vi "AlliGator Calibrated Phasor Maps Series Script.vi"(0 "Alligator Queue Elements in":T2[](array[typedef]), 1 "Calibration Map/Gate Step List":T1[](array[typedef]), 2 "Destination Folder":path, 3 "File Suffix (# Steps will be added)":string caption="File Name (# Steps will be added)", 4 "Save Phasor Plot":bool, 5 "Error In":errorcluster, 6 "Phasor Graph refnum":refnum<vi>) -> (14 "Alligator Queue Elements out":T2[](array[typedef]), 17 "Message":string, 19 "Error Out":errorcluster)   [LabVIEW 2021, in "AlliGator Scripts.lvlib"]
doc: "Loops through a series of FLI Dataset files, loads them with the specified gate step, and performs an All ROIs Phasor Analysis, using the resulting phasor plot as Phasor Calibration Map. This map is then save and optionally, the phasor plot as well."
uses:
  AlliGator Scripts.lvlib
  Action Engine/AlliGator Q Element.ctl
  Action Engine/AlliGator Q Event.ctl
  AlliGator Dataset + Calibration Map + Gate Step.ctl
  Globals, Variables, Constants/AlliGator Variables List.ctl
  Action Engine/Alligator Elements Order in Action Stack.ctl
  Graphs/XY Graph/XY Graph Mouse Click Event Data.ctl
  Graphs/XY Graph/XY Graph Refnum.ctl
  <vilib>/Utility/miscctls.llb/LVPoint32TypeDef.ctl
  Graphs/XY Graph/XY Graph New Plot Name Data.ctl
  Files/Load-Save File Info.ctl
  Action Engine/AlliGator Add Single Action to Stack.vi
  Action Engine/AlliGator Add Action Array to Stack.vi
  Action Engine/AlliGator Action Engine.lvlib
  Strings/Strings.lvlib
  Files/AlliGator Files.lvlib
  Globals, Variables, Constants/AlliGator Globals, Variables & Constants.lvlib
  Graphs/XY Graph/XY Graph Add-Ons.lvlib
  Files/Files.lvlib
panel:
  out "Series Length":i32
  # "see the AlliGator License on the block diagram (Ctrl+E or Window:Show Block Diagram)"
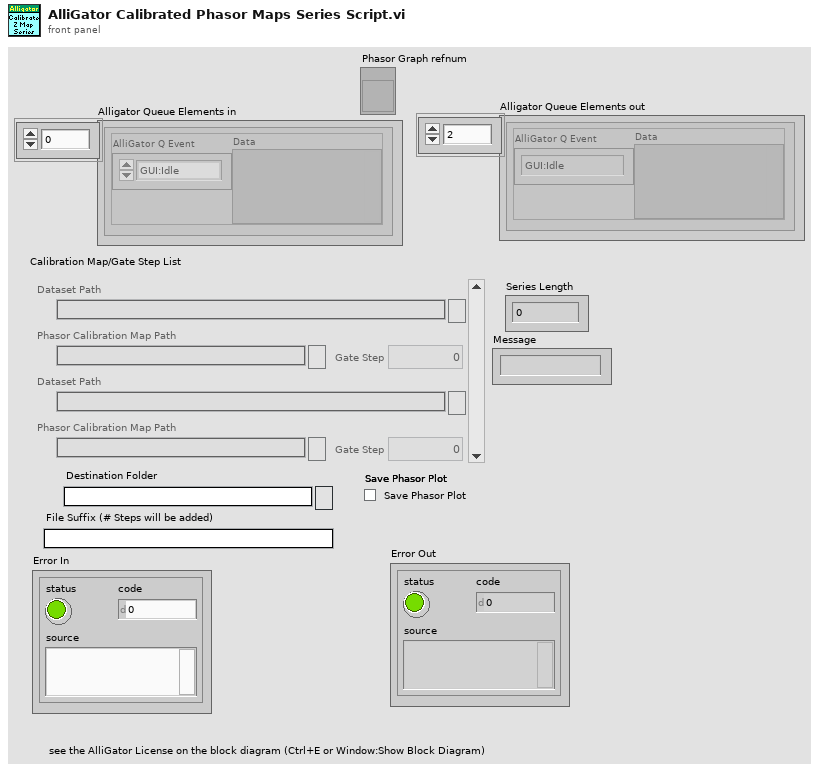
[diagram p1: front panel]
types:
  T1 = typedef "AlliGator Scripts.lvlib/AlliGator Dataset + Calibration Map + Gate Step.ctl" = cluster{"Phasor Calibration Map Path":path, "Gate Step":i32, "Dataset Path":path}
  T2 = typedef "AlliGator Action Engine.lvlib/AlliGator Q Element.ctl" = cluster{"AlliGator Q Event":T3, "Data":variant}
  T3 = typedef "AlliGator Action Engine.lvlib/AlliGator Q Event.ctl" = enum16{"---- Files ----", "Files:Set Batch Export Files To Save", "Files:Set Dataset Loading & Pre-processing Options", "Files:Check #Frames in Dataset", "Files:Increment Frame Index", "Files:Open Mask Image", "Files:Open White Light Image", "Files:Open Single Dataset", "Files:New Folder of Folders Selected", "Files:Load File (all Types)_Scriptable", "Files:Move Flattened Series to Folders Series", "Files:Select Folder", "Files:Load FLI Dataset", "Files:Load Swiss SPAD 1 Dataset", "Files:Load Swiss SPAD 2 Dataset", "Files:Load .sdt FLI Dataset", "Files:Load .ptu FLI Dataset", "Files:Load .bin FLI Dataset", "Files:Load Single Gate Image Folder", "Files:Load I/m/phi Dataset (deprecated)", "Files:Load Single Image", "Files:Subtract Background File", "Files:Export FLI Dataset", "Files:Load HDF5 FLI Dataset", "Files:Set Destination File Path", "Files:Save Mask Image", "Files:Batch Conversion", "Files:New Folder Selected", "Files:Close FLI Dataset", "Files:Close FLI Dataset Series", "Files:Close White Light Image", "Files:Close Mask Image", "---- FLI Dataset ----", "FLI Dataset:Channel Arithmetic", "FLI Dataset:Export Average Lifetime Map as ASCII", "FLI Dataset:Export User-Defined Quantity Map as ASCII", "FLI Dataset:Python Function FLI Dataset Event", "FLI Dataset:ROI Analysis", "FLI Dataset:Tilted Logistic Square Gated IRF Characteristics Map", "FLI Dataset:Logistic Square Gated IRF Characteristics Map", "FLI Dataset:Square Gated IRF Characteristics Map", "FLI Dataset:Multi-ROI Single-Pixel Phasor Analysis", "FLI Dataset:Multi-ROI Single-Pixel NLSF Analysis", "FLI Dataset:All ROIs IRF Extraction", "FLI Dataset:All ROIs Decay Fit Non-Interactive (Fast + Individual IRF)", "FLI Dataset:All ROIs Phasor Analysis", "FLI Dataset:All ROIs Decay Fit", "FLI Dataset:Fluorescence Decay Statistics", "FLI Dataset:Update Decay Statistics Graph", "FLI Dataset:Get Decay from ROI", "FLI Dataset:All ROIs Average Lifetimes", "---- FLI Dataset Series ----", "FLI Dataset Series:Sum All Datasets in Series", "FLI Dataset Series:Add Dataset to Accumulated Dataset", "FLI Dataset Series:Display Accumulated Dataset", "FLI Dataset Series:Clear Dataset Series Sum", "FLI Dataset Series:Time-Series Analysis (NLSF)", "FLI Dataset Series:Time-Series Analysis (Phasor)", "---- Image ----", "Image:Update Image Profile Plots", "Image:Image Histogram Cursor Move", "Image:Image Histogram", "Image:Image Contrast", "Image:Set Image Histogram Cursor Move Flag", "Image:Clear Image Overlay", "Image:Use ROI as Search Area", "Image:Set ROI Diameter", "Image:Save Image Data as TIFF", "Image:Save Displayed Image with Overlay", "Image:Save Image Overlay Only", "Image:Save Image as Hot Pixel Mask", "Image:Change Source Image Color Palette", "Image:Copy Image to Clipboard", "Image:Source Image ROI Selection", "Image:Delete All ROIs", "Image:Delete All Unselected ROIs", "Image:Delete ROI", "Image:Merge All ROIs", "Image:Store ROI", "Image:Source Image ROI Storage", "Image:Export ROI Description to Notebook", "Image:Save ROI", "Image:Load ROI", "Image:Paste ROI Definition", "Image:Clear ROI", "Image:Identify ROIs in Mask Image", "Image:Create Complementary ROI", "Image:Create Contour ROI", "Image:Create ROI(s) from Pixels with Peak above Min_Scriptable", "Image:Create ROI(s) from Pixels with Intensity above Min_Scriptable", "Image:Compute ROI Statistics", "Image:Delete ROI(s) based on ROI Characteristics", "Image:Create ROI Grid", "Image:ROI to Individual Pixel ROIs", "Image:Python Function Source Image Event", "Image:Show Phasor Calibration Map ROI Centers", "Image:Convert ROI to Mask Image", "Image:Mouse Move", "Image:Mouse Up", "Image:Set Source Image Mouse Move Flag", "Image:Add Scale Bar Overlay", "Image:Delete Existing ROIs Option", "Image:Overlay ROI Median", "Image:Check Current ROI", "---- Decay ----", "Decay:Clear IRF/Reference Plot", "Decay:Clear Local IRFs", "Decay:Add Decay to Graph", "Decay:Smoothen Plot", "Decay:Smoothen Plot Tail", "Decay:Average Selected Plots", "Decay:Extract IRF", "Decay:Optimal IRF Extraction", "Decay:Threshold IRF", "Decay:Fit to Model IRF", "Decay:Fit IRF to Square Gate", "Decay:Fit IRF to Logistic Square Gate", "Decay:Fit IRF to Tilted Logistic Square Gate", "Decay:Create Bounding Cursors Set", "Decay:Export Bounding Cursors Definition to Notebook", "Decay:Denoise Plot", "Decay:Compute Cumulative Function", "Decay:Use as Reference Decay", "Decay:Show Reference Decay/IRF", "Decay:Extrapolate Decay", "Decay:Create Head & Tail Bounding Cursors", "Decay:Store Cursor-defined Head & Tail Fractions", "Decay:Rebin Plot", "Decay:1-Normalize Decay", "Decay:[0-1]-Normalize Plot", "Decay:Straighten Decay", "Decay:Shift Decay", "Decay:Fold Decay", "Decay:Fit Decay", "Decay:Global Fit of Selected Decays", "Decay:Post Global Fit Script", "Decay:Add Global Fit Parameters to Graph", "Decay:Add Decay Parameter(s) to Plot (Graph)", "Decay:Export Decay to Phasor Graph", "Decay:Plot Decay Shifts", "Decay:Compute Average Lifetime", "Decay:Plot Convolution", "Decay:Graph Tip Strip Update", "---- Decay Statistics ----", "Decay Statistics:Tip Strip Update", "---- Intensity Time Trace ----", "Intensity Time Trace:Use File Timestamp", "Intensity Time Trace:Load Intensity Corrections File", "Intensity Time Trace:Clear Intensity Corrections File", "Intensity Time Trace:Tip Strip Update", "---- Phasor Plot ----", "Phasor Plot:Build Phasor Plot", "Phasor Plot:Change Phasor Plot Color Palette", "Phasor Plot:Adjust Phasor Plot Display Range", "Phasor Plot:Highlight Image ROI in Phasor Plot", "Phasor Plot:Save Phasor Plot Image with Overlay", "Phasor Plot:Export Complex Phasor Map", "Phasor Plot:Export Phasor Ratio Map", "Phasor Plot:Export Average Lifetime Map", "Phasor Plot:Compute Phase Lifetime Histogram", "Phasor Plot:Compute Phasor Ratio Histogram", "Phasor Plot:Compute Phase Lifetime vs Intensity Scatter Plot", "Phasor Plot:Weber 2-Component Decomposition", "Phasor Plot:Update Phasor Color Map Vertices", "Phasor Plot:Clear Phasor Overlay", "Phasor Plot:Use Segment Extremities as References", "Phasor Plot:Use UC/Segment Intersections as References", "Phasor Plot:Use UC/Principal Axis Intersections as References", "Phasor Plot:Use UC/Linear Fit Intersections as References", "Phasor Plot:Update Phasor Plot Reference", "Phasor Plot:Show Local Phasor Info in Phasor Plot", "Phasor Plot:Update Phasor Plot State", "Phasor Plot:Phasor Plot ROI Storage", "Phasor Plot:Phasor Plot ROI Selection", "Phasor Plot:Python Function Phasor Plot Event", "Phasor Plot:Overlay Phasor ROI, Ratio or Map in Source Image", "Phasor Plot:Compute Decay of Selected Phasors", "Phasor Plot:Phasor at Image Pixel", "Phasor Plot:Mouse Move", "Phasor Plot:Mouse Up", "Phasor Plot:Display Range Mouse Move", "Phasor Plot:Set Mouse Move Flag", "---- Phasor Graph ----", "Phasor Graph:Calibrated Phasor Map Series", "Phasor Graph:Whole Image Phasor Scatter Plot (deprecated)", "Phasor Graph:Get Phasor Value", "Phasor Graph:Create New Phasor Plot Dialog", "Phasor Graph:Update Last Phasor Value", "Phasor Graph:Update Phasor (m, phi)", "Phasor Graph:Remove Single Phasor from Plot", "Phasor Graph:Add Single Phasor to Plot", "Phasor Graph:Remove Phasor Plot", "Phasor Graph:Remove Selected Phasor Plots", "Phasor Graph:Clear Phasor Data", "Phasor Graph:Clear Phasor Graph", "Phasor Graph:Cursor Move", "Phasor Graph:Draw Cursor Connecting Line", "Phasor Graph:Clear Cursor Connecting Line", "Phasor Graph:Find UC Intersection", "Phasor Graph:Use UC/Cursor-Defined Line Intersections", "Phasor Graph:Use Selected Plots Fitted Line/UC Intersections", "Phasor Graph:Use Selected Plots Principal Axis/UC Intersections", "Phasor Graph:Show Single Phasor", "Phasor Graph:Save Single Phasor Plot", "Phasor Graph:Save All Phasor Plots", "Phasor Graph:Load Phasor Plot(s)", "Phasor Graph:Phasor Multiplication", "Phasor Graph:Compute Average Phasor", "Phasor Graph:Compute Multiple Average Phasors (Selected Plots)", "Phasor Graph:Export Single Phasor Plot Phase Lifetimes", "Phasor Graph:Phase Lifetime Trajectory", "Phasor Graph:Phase Lifetime vs Intensity Scatter Plot (deprecated)", "Phasor Graph:Parameter 2 vs Parameter 1 Scatter Plot", "Phasor Graph:Use Cursor n Location", "Phasor Graph:Set Reference n to Current Phase Lifetime Value", "Phasor Graph:Set Reference n to Lifetime Value", "Phasor Graph:Set Cursor n Location", "Phasor Graph:Save Phasor Graph Image", "Phasor Graph:Update SEPL Plot", "Phasor Graph:Export Single Phasor Plot Data", "Phasor Graph:Export Selected Phasor Plots Data", "Phasor Graph:Python Function Phasor Graph Event", "Phasor Graph:Tip Strip Update", "---- Calibration ----", "Calibration:Set Calibration Type", "Calibration:Load/Save Phasor Calibration", "Calibration:Load/Save Phasor Calibration Series", "Calibration:Load/Save Phasor Calibration Map", "Calibration:Use as Calibration", "Calibration:Compute Optimal Calibration from Phasor References", "Calibration:Clear Phasor Calibration", "Calibration:Single Phasor Calibration Information", "Calibration:Use as Calibration Series", "Calibration:Use as Calibration Map", "Calibration:Clear Calibration Series", "Calibration:Phasor Calibration Series Information", "Calibration:Clear Calibration Map", "Calibration:Phasor Calibration Map Information", "Calibration:Apply Phasor Calibration", "Calibration:Update Single Plot Calibration", "Calibration:Update Multiple Plots Calibration", "Calibration:Clear Single Plot Calibration", "Calibration:Clear All Plots Calibrations", "Calibration:Clear Plot(s) Calibration(s)?", "Calibration:Phasor Calibration Maps (# Gates Series)", "---- Phasor Ratio ----", "Phasor Ratio:Clear Reference n", "Phasor Ratio:Toggle Selected Plot(s)  Lock to Reference 1", "Phasor Ratio:Use as Reference n", "Phasor Ratio:Send Reference n to Notebook", "Phasor Ratio:Toggle Selected Plot(s)  Lock to Reference 2", "Phasor Ratio:Compute Phasor Ratio at Mouse Location", "Phasor Ratio:Compute Phasor Plot's Average Phasor Ratio", "Phasor Ratio:Compute Time-Series Phasor Ratios", "Phasor Ratio:Fit Line to Phasor Ratio Plot", "Phasor Ratio:Save References", "Phasor Ratio:Load References", "Phasor Ratio:Update Phasor Reference 1", "Phasor Ratio:Update Phasor Reference 2", "Phasor Ratio:Move Cursor n to Reference n", "Phasor Ratio:Use as Phasor Reference 1 Lifetime", "Phasor Ratio:Use as Phasor Reference 2 Lifetime", "Phasor Ratio:Export Phasor Ratio Map as ASCII", "Phasor Ratio:Tip Strip Update", "---- Lifetime & Other Parameters Graph ----", "Lifetime:Tip Strip Update", "---- Decay Fit Parameter Map ----", "Decay Fit Parameter Map:Export ROI NLSF Data as ASCII", "Decay Fit Parameter Map:Set Decay Fit Parameter Map Selection", "Decay Fit Parameter Map:Build Decay Fit Parameter Map", "Decay Fit Parameter Map:Change Decay Fit Parameter Map Color Palette", "Decay Fit Parameter Map:Export Decay Fit Parameter Map Data as ASCII", "Decay Fit Parameter Map:Export All Decay Fit Parameter Maps Data as ASCII", "Decay Fit Parameter Map:Selected Parameter Scatterplot", "Decay Fit Parameter Map:Parameter 2 vs Parameter 1 Scatterplot", "Decay Fit Parameter Map:Save Decay Fit Parameter Map Image", "Decay Fit Parameter Map:Save-Load IRFs & Fit Data", "Decay Fit Parameter Map:Update Local Decay Plots", "Decay Fit Parameter Map:Python Function Decay Fit Parameters Map Event", "Decay Fit Parameter Map:Overlay Decay Fit Parameter Map in Source Image", "Decay Fit Parameter Map:Selected Parameter vs Intensity Scatterplot", "Decay Fit Parameter Map:Mouse Up", "Decay Fit Parameter Map:Display Range Mouse Move", "---- Parameter Map ----", "Parameter Map:Export ROI Parameters Data as ASCII", "Parameter Map:Delete Parameter Map Set", "Parameter Map:Update Parameter List", "Parameter Map:Build Parameter Map", "Parameter Map:Change Parameter Map Color Palette", "Parameter Map:Export Parameter Map Data as ASCII", "Parameter Map:Export All Parameter Maps Data as ASCII", "Parameter Map:Selected Parameter Scatterplot", "Parameter Map:Parameter 2 vs Parameter 1 Scatterplot", "Parameter Map:Selected Parameter vs Intensity Scatterplot", "Parameter Map:Save Parameter Map Image", "Parameter Map:Save-Load IRFs & Parameter Maps (TODO)", "Parameter Map:Set Parameter Map Selection", "Parameter Map:Python Function Parameter Map Event", "Parameter Map:Overlay Parameter Map in Source Image", "Parameter Map:Update Local Decay Plots", "Parameter Map:Mouse Up", "Parameter Map:Display Range Mouse Move", "---- Generic Graph ----", "Generic Graph:Generic XY Graph Event", "Generic Graph:Python Function XY Graph Event", "Generic Graph:New Plot", "Generic Graph:Save Plot", "Generic Graph:XY Plot Histogram", "Generic Graph:Set XY Graph Plot Name", "Generic Graph:Set Last Cursor Style", "Generic Graph:Tip Strip Update", "---- GUI ----", "GUI:Start Script", "GUI:Type of Displayed Image Changed", "GUI:Gate Image Slide Changed", "GUI:Show Busy Icon", "GUI:Show Busy Icon & Abort Button", "GUI:Hide Busy Icon", "GUI:Hide Busy Icon & Abort Button", "GUI:Abort", "GUI:End Script", "GUI:Start Timing", "GUI:End Timing", "GUI:Set State Indicator", "GUI:Send Parameters JSON Strings to Clipboard", "GUI:Set Gate Step", "GUI:Idle", "GUI:Initialization", "GUI:Quit", "GUI:Increment Dataset Index", "GUI:Set Dataset Index to -1", "GUI:Time Series Slider Moved", "GUI:Time Series Slider Changed", "GUI:Toggle Playback or Loop", "GUI:Playback Script", "GUI:Set Phasor Frequency", "GUI:Open Window", "GUI:Start Test Script", "GUI:End Test Script", "DEBUG"}
  T4 = typedef "AlliGator Globals, Variables & Constants.lvlib/AlliGator Variables List.ctl" = enum16{"---- GUI ----", "GUI:Initialization Status", "GUI:State Indicators Refnum", "GUI:Original AlliGator Menu Items", "GUI:Current Action Loop State", "GUI:Script in progress", "GUI:Playback", "GUI:Loop Playback", "GUI:Search ROI Used", "GUI:Search ROI", "Decay Graph Max Legend Size", "Intensity Graph Max Legend Size", "Decay Statistics Graph Max Legend Size", "Phasor Graph Max Legend Size", "Phasor Ratio Graph Max Legend Size", "Lifetime Graph Max Legend Size", "---- Files ----", "Files:Export Dataset Frames as Individual Files", "Files:Show Batch Export Help Balloons", "Files:Frames in Dataset", "Files:ptu File Frame Start Indices", "Files:Current Frame in Dataset", "Files:Current Frame Timestamp", "Files:Dataset Loaded", "Files:Dataset Metadata", "Files:Dataset Channel", "Files:Dataset Data Description", "Files:Background Dataset Metadata", "Files:Background Dataset Channel", "Files:Background Dataset Data Description", "Files:Background File Subtraction", "Files:Background File Path", "Files:Background File Pile-up Correction", "Files:Background File Pixel Well Capacity", "Files:Background File Scaling Factor", "Files:Current Dataset Load Settings", "Files:Dataset Path", "Files:ICCD-specific Information", "Files:Macrotime Gate Separation", "------ Python Plugins ------", "Python Plugins:Information", "Python Plugins:Python Session", "Python Plugins:Valid Python Session?", "---- Source Image ----", "Source Image:ROIs", "Source Image:Current ROI", "Source Image:ROI Event Refnum", "X_Source Image Display Range", "X_Source Image Palette Information", "X_Type of Displayed Image", "X_Time Gate Slider", "Source Image:Palette List", "Source Image:Scale", "Source Image:ROI Overlay Color", "Source Image:Overlay to Erase", "Source Image:Is Displayed Image Accumulated", "Source Image:White Light Image Modified", "Source Image:Mask Image Modified", "---- Image Profile Window ----", "Image Profile:Window Event Refnum", "Image Profile:IntensityType", "Image Profile:Intensity Average Type", "Image Profile:Intensity-weighted SDV", "Image Profile:Box Profile Type", "Image Profile:Window Open", "Image Profile:Plotted Fit Parameter", "------ Phasor Graph -------", "Phasor Graph:Show Line", "---- Phasor Plot ---", "Phasor Plot:Parameters Changed", "Phasor Plot:FLI Dataset Modified since last Calculation", "Phasor Harmonics Data", "Selected Phasor Harmonics", "Phasor Harmonic Manager Event Refnum", "Phasor Plot:ROIs", "Phasor Plot:Current ROI", "Phasor Plot:ROI Event Refnum", "Phasor Plot:Image Reference Points", "Phasor Plot:Computed", "Phasor Plot:Palette Information", "Phasor Plot:Palette List", "Phasor Plot:Phasor Ratio Palette Information", "Phasor Plot:Phasor Ratio Palette List", "Phasor Plot:Image Scale", "Phasor Plot:Image Overlay to Erase", "Phasor Plot:Image Elements to Update", "Phasor Plot:Current Calculation Parameters", "Phasor Plot:Current Calibration Options", "Phasor Plot:Reset Cumulated Phasor Plot", "Phasor Plot:Reference 1", "Phasor Plot:Lifetime Reference 1", "Phasor Plot:Reference 1 Frequency", "Phasor Plot:Reference 2", "Phasor Plot:Lifetime Reference 2", "Phasor Plot:Reference 2 Frequency", "---- Decay Analysis ----", "Number of Selected Decays to Fit", "LS Fit Results", "LAR Fit Results", "BS Fit Results", "Last Decay Max - Min", "Best Fit Parameters", "Best Fit Parameter Names", "Actual Size X", "Actual Size Y", "Binning X", "Binning Y", "Actual # Gates", "Dataset Number", "Gates to...", "Gates Skipped", "Gates to keep", "Gate Step", "Gate Separation", "Reversed Gates", "Pile-up Correction", "Pixel Well Capacity", "Background Subtracted", "Background Subtraction Method", "Background Definition Range", "Background File (deprecated)", "Number of Dataset Accumulated", "Array of Accumulated Dataset Paths", "Do Averaged Datasets", "Destination File Path", "Process Plot Target", "Use 1/D as Phasor Frequency", "---- Decay Fit Parameter Map -----", "Decay Fit Parameter Map:Palette Information", "Decay Fit Parameter Map:Palette List", "---- Parameter Map ----", "Parameter Map:Palette Information", "Parameter Map:Palette List", "------- Local Decay Window ---------", "Local Decay Graph Window:Event Refnum", "Local Decay Graph Window:Use normalized IRF for convolution", "----- Miscellaneous ----", "Misc:Skippable Dialog Windows Status"}
  T5 = enum16{"Start Script", "Load & Analyze Data", "End Script"}
  T6 = typedef "AlliGator Action Engine.lvlib/Alligator Elements Order in Action Stack.ctl" = enum16{"Enqueue 2 AFTER 1", "Enqueue 2 BEFORE 1"}
  T7 = typedef "Files.lvlib/Load-Save File Info.ctl" = cluster{"Load/Save":bool, "File Path":path}
  T8 = typedef "XY Graph Add-Ons.lvlib/XY Graph New Plot Name Data.ctl" = cluster{"XY Graph Refnum":T9, "Plot Index":i32, "Plot Name":string, "Allow Duplicate":bool}
  T9 = typedef "XY Graph Add-Ons.lvlib/XY Graph Refnum.ctl" = refnum<vi>
  T10 = typedef "XY Graph Add-Ons.lvlib/XY Graph Mouse Click Event Data.ctl" = cluster{"Multiplot XY Graph":T9, "Mouse Coordinates":T11}
  T11 = typedef "LVPoint32TypeDef.ctl" = cluster{"Horizontal":i32, "Vertical":i32}
  T12 = cluster{"Mouse Click Event Data":T10, "Save as...":bool}
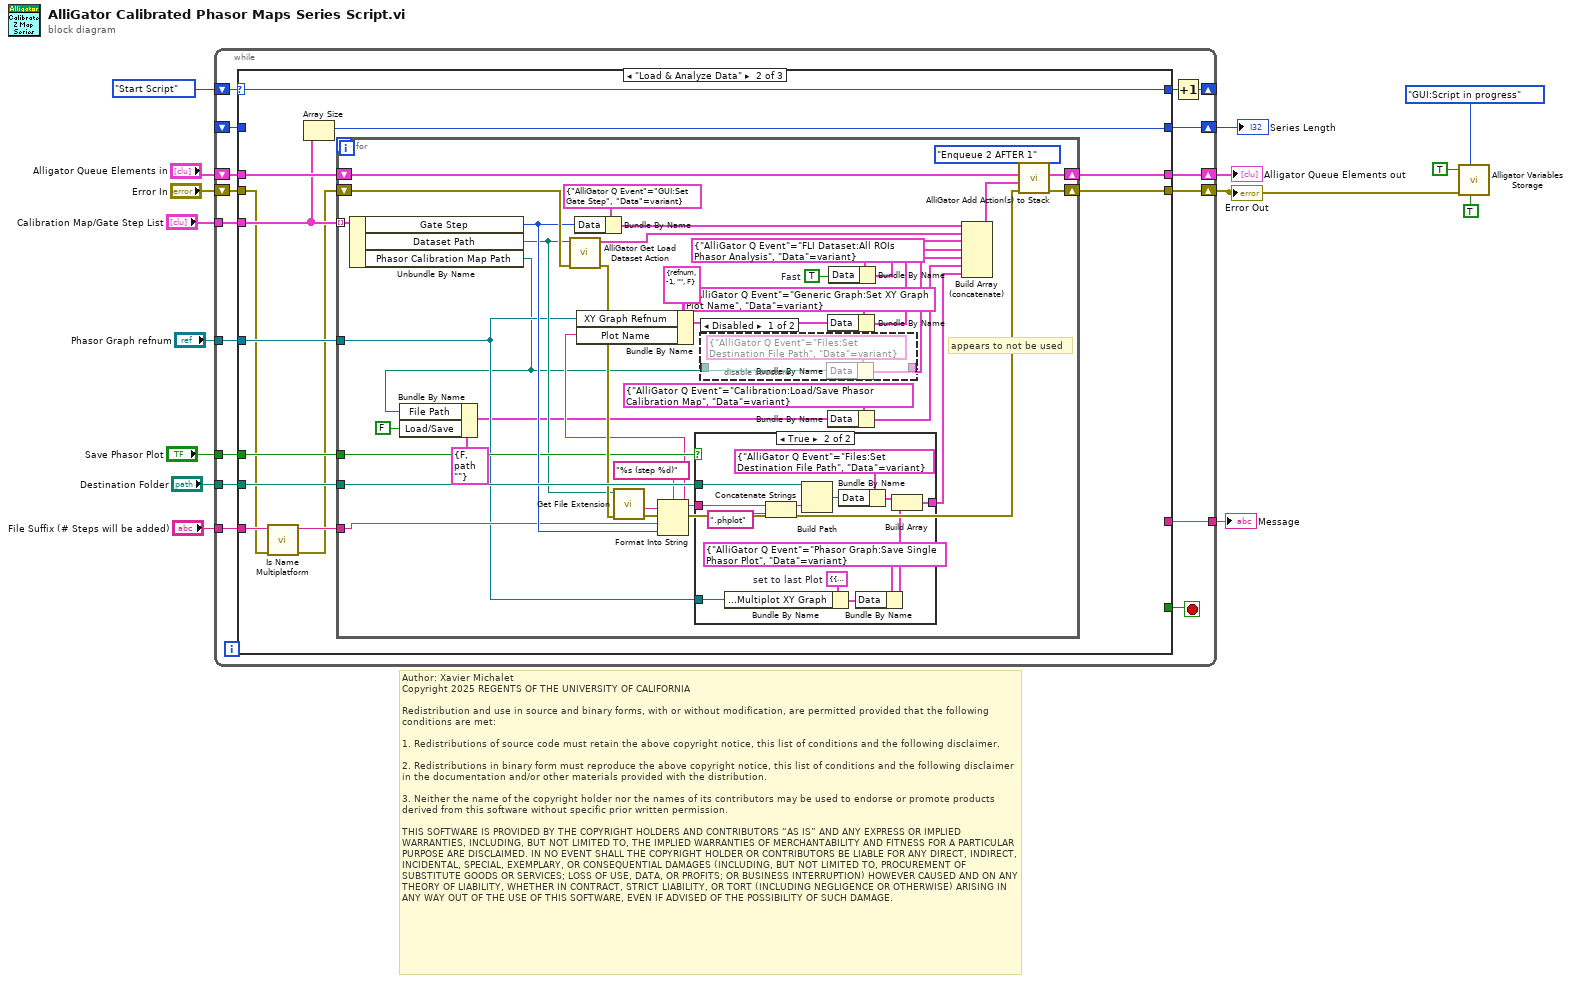
[diagram p0: block diagram]
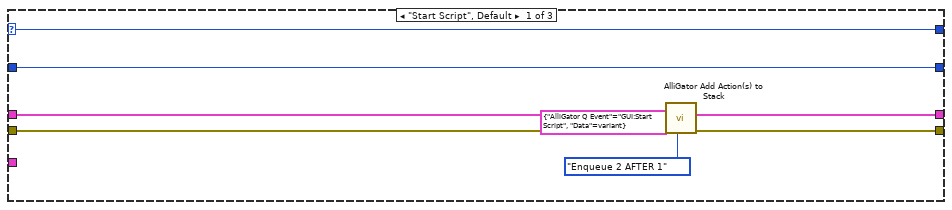
[diagram p2: hidden frame]
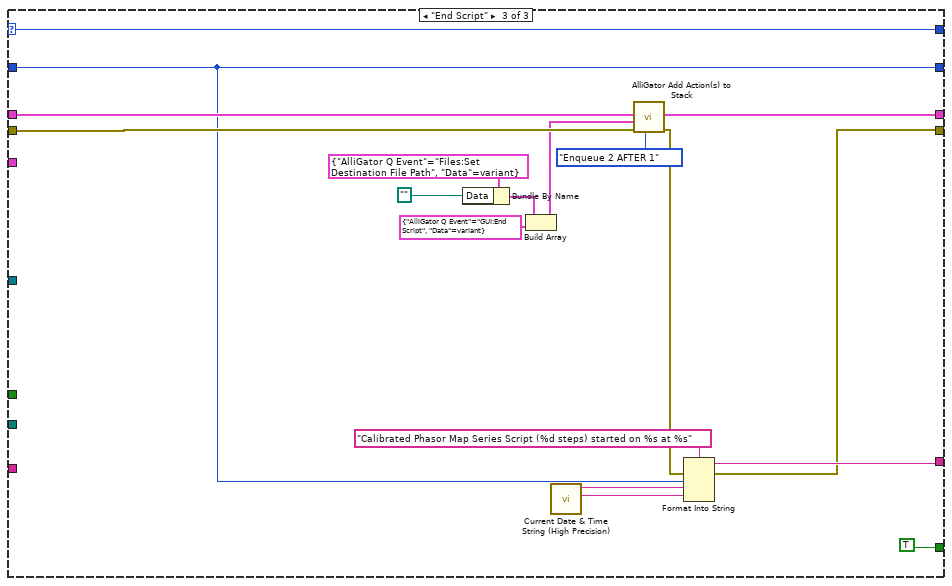
[diagram p5: hidden frame]
diagram:
  # "Author: Xavier Michalet\nCopyright 2025 REGENTS OF THE UNIVERSITY OF CALIFORNIA\n\nRedistribution and use in source and binary forms, with or without modification, are permitted provided that the following conditions are met:\n\n1. Redistributions of source code must retain the above copyright notice, this list of conditions and the following disclaimer.\n\n2. Redistributions in binary form must reproduce the above copyright notice, this list of conditions and the following disclaimer in the documentation and/or other materials provided with the distribution.\n\n3. Neither the name of the copyright holder nor the names of its contributors may be used to endorse or promote products derived from this software without specific prior written permission.\n\nTHIS SOFTWARE IS PROVIDED BY THE COPYRIGHT HOLDERS AND CONTRIBUTORS “AS IS” AND ANY EXPRESS OR IMPLIED WARRANTIES, INCLUDING, BUT NOT LIMITED TO, THE IMPLIED WARRANTIES OF MERCHANTABILITY AND FITNESS FOR A PARTICULAR PURPOSE ARE DISCLAIMED. IN NO EVENT SHALL THE COPYRIGHT HOLDER OR CONTRIBUTORS BE LIABLE FOR ANY DIRECT, INDIRECT, INCIDENTAL, SPECIAL, EXEMPLARY, OR CONSEQUENTIAL DAMAGES (INCLUDING, BUT NOT LIMITED TO, PROCUREMENT OF SUBSTITUTE GOODS OR SERVICES; LOSS OF USE, DATA, OR PROFITS; OR BUSINESS INTERRUPTION) HOWEVER CAUSED AND ON ANY THEORY OF LIABILITY, WHETHER IN CONTRACT, STRICT LIABILITY, OR TORT (INCLUDING NEGLIGENCE OR OTHERWISE) ARISING IN ANY WAY OUT OF THE USE OF THIS SOFTWARE, EVEN IF ADVISED OF THE POSSIBILITY OF SUCH DAMAGE."
  n1 = while {
    shift-right: [w28] -> w6
    shift-left: "Error In" -> [w31]
    shift-right: [w26] -> _
    shift-left: T5."Start Script" -> [w29]
    shift-right: [w24] -> w12
    shift-left: "Alligator Queue Elements in" -> [w30]
    tunnel: "Calibration Map/Gate Step List" -> [w23]
    tunnel: "Destination Folder" -> [w22]
    tunnel: "File Suffix (# Steps will be added)" -> [w21]
    shift-right: [w20] -> w9
    shift-left: _ -> [w19]
    tunnel: "Phasor Graph refnum" -> [w18]
    tunnel: "Save Phasor Plot" -> [w17]
    tunnel: [w16] -> w1
    stop <- w25 stop-if-true
    n2 = case shown="\"Load & Analyze Data\"" w29 {
      selector: w29 -> [w39 w51 w122]
      tunnel: w31 -> [w36 w40 w119]
      tunnel: w30 -> [w34 w52 w120]
      tunnel: [w37 w49 w106] -> w28
      tunnel: [w39 w51 w122] -> w27
      tunnel: [_ _ TRUE] -> w25
      tunnel: [w35 w50 w117] -> w24
      tunnel: w23 -> [_ w43 _]
      tunnel: w22 -> [_ w48 _]
      tunnel: w21 -> [_ w47 _]
      tunnel: [w38 w45 w109] -> w20
      tunnel: w19 -> [w38 _ w109]
      tunnel: w18 -> [_ w44 _]
      tunnel: w17 -> [_ w42 _]
      tunnel: [_ _ w108] -> w16
      frame "Start Script", Default {
        n3 = call-poly "AlliGator Add Action(s) to Stack.vi"("Elements Order in Action Stack (Default: 2 BEFORE 1)"=Alligator_Elements_Order_in_Action_Stack."Enqueue 2 AFTER 1", "Error In"=w36, "Alligator Atomic Action"=T2 {"AlliGator Q Event"=enum."GUI:Start Script", "Data"=variant}, "Alligator Queue Element 1"=w34) -> ("Error Out"=w37:errorcluster, "Alligator Queue Element 1 (+ 2)"=w35:T2[])  [unwired: 6 in]
      }
      frame "Load & Analyze Data" {
        n4 = call <vilib>:"Is Name Multiplatform.vi"("error in (no error)"=w40, "filename"=w47) -> ("error out"=w41:errorcluster, "suggested filename"=w46:string)  [unwired: 5 in, 3 out]
        n5 = Array Size(array=w43) -> (size(s)=w45:i32)
        n6 = for {
          shift-right: [w89] -> w50
          shift-left: w52 -> [w85]
          shift-right: [w88] -> w49
          shift-left: w41 -> [w82]
          tunnel: w43 -> [w77] mode=indexing
          tunnel: w46 -> [w63]
          tunnel: w48 -> [w86]
          tunnel: w44 -> [w58]
          tunnel: w42 -> [w75]
          w71 = TRUE  # Fast
          # "appears to not be used"
          n7 = Unbundle By Name(w77) -> ("Gate Step"=w76:i32, "Dataset Path"=w73:path, "Phasor Calibration Map Path"=w53:path)
          n8 = Bundle By Name(cluster=T7 {"Load/Save"=FALSE, "File Path"=path ""} ("Calibration File Information"), "File Path"=w53, "Load/Save"=FALSE) -> (w54:T7)
          n9 = call "AlliGator Get Load Dataset Action.vi"("Error In"=w82, "File/Folder Path"=w73) -> ("Error Out"=w81:errorcluster, "Alligator Atomic Action"=w80:T2)  [unwired: 8 in]
          n10 = Bundle By Name(cluster=T2 {"AlliGator Q Event"=enum."GUI:Set Gate Step", "Data"=variant} ("element"), "Data"=w76) -> (w84:T2)
          n11 = call <vilib>:"Get File Extension.vi"("error in (no error)"=w81, "file"=w73) -> ("error out"=w65:errorcluster, "filename without extension"=w66:string)  [unwired: 5 in, 3 out]
          n12 = Format Into String(format string="%s (step %d)", initial string=w66, error in=w65, w63, w76) -> (resulting string=w57:string, error out=w62:errorcluster)
          n13 = Bundle By Name(cluster=T8 {"XY Graph Refnum"=refnum, "Plot Index"=-1, "Plot Name"="", "Allow Duplicate"=FALSE} ("New Plot Name Data"), "XY Graph Refnum"=w58, "Plot Name"=w57) -> (w60:T8)
          n14 = case shown="True" w75 {
            tunnel: w86 -> [_ w105]
            tunnel: [_ w101] -> w74
            tunnel: w58 -> [_ w96]
            tunnel: w57 -> [_ w95]
            frame False {
            }
            frame True {
              w98 = T12 {"Mouse Click Event Data"={"Multiplot XY Graph"=refnum, "Mouse Coordinates"={"Horizontal"=2147483647, "Vertical"=0}}, "Save as..."=FALSE}  # set to last Plot
              n15 = Bundle By Name(cluster=w98, "Mouse Click Event Data.Multiplot XY Graph"=w96) -> (w97:T12)
              n16 = Concatenate Strings(w95, ".phplot" ("string")) -> (w94:string)
              n17 = Build Path(base path=w105, name or relative path=w94) -> (appended path=w102:path)
              n18 = Bundle By Name(cluster=T2 {"AlliGator Q Event"=enum."Files:Set Destination File Path", "Data"=variant} ("element"), "Data"=w102) -> (w103:T2)
              n19 = Bundle By Name(cluster=T2 {"AlliGator Q Event"=enum."Phasor Graph:Save Single Phasor Plot", "Data"=variant} ("element"), "Data"=w97) -> (w99:T2)
              n20 = Build Array(w103, w99) -> (w101:T2[])
            }
          }
          n21 = disable-structure shown="Disabled" {
            disable-tunnel: [w91 _] -> w68
            disable-tunnel: w53 -> [w90 _]
            frame Disabled {
              n22 = Bundle By Name(cluster=T2 {"AlliGator Q Event"=enum."Files:Set Destination File Path", "Data"=variant} ("element"), "Data"=w90) -> (w91:T2)
            }
            frame Enabled {
            }
          }
          n23 = Bundle By Name(cluster=T2 {"AlliGator Q Event"=enum."Generic Graph:Set XY Graph Plot Name", "Data"=variant} ("element"), "Data"=w60) -> (w59:T2)
          n24 = Bundle By Name(cluster=T2 {"AlliGator Q Event"=enum."Calibration:Load/Save Phasor Calibration Map", "Data"=variant} ("element"), "Data"=w54) -> (w70:T2)
          n25 = Bundle By Name(cluster=T2 {"AlliGator Q Event"=enum."FLI Dataset:All ROIs Phasor Analysis", "Data"=variant} ("element"), "Data"=w71) -> (w69:T2)
          n26 = Build Array (concatenate)(w84, w80, w69, w59, w68, w70, w74) -> (w83:T2[])
          n27 = call-poly "AlliGator Add Action(s) to Stack.vi"("Elements Order in Action Stack (Default: 2 BEFORE 1)"=Alligator_Elements_Order_in_Action_Stack."Enqueue 2 AFTER 1", "Error In"=w62, "Alligator Queue Element 2"=w83, "Alligator Queue Element 1"=w85) -> ("Error Out"=w88:errorcluster, "Alligator Queue Element 1 (+ 2)"=w89:T2[])  [unwired: 6 in]
        }
      }
      frame "End Script" {
        n28 = Bundle By Name(cluster=T2 {"AlliGator Q Event"=enum."Files:Set Destination File Path", "Data"=variant} ("element"), "Data"=path "") -> (w111:T2)
        n29 = Build Array(w111, T2 {"AlliGator Q Event"=enum."GUI:End Script", "Data"=variant} ("element")) -> (w113:T2[])
        n30 = call "Current Date & Time String (High Precision).vi"() -> ("time string"=w115:string, "date string"=w114:string)  [unwired: 8 in, 2 out]
        n31 = call-poly "AlliGator Add Action(s) to Stack.vi"("Elements Order in Action Stack (Default: 2 BEFORE 1)"=Alligator_Elements_Order_in_Action_Stack."Enqueue 2 AFTER 1", "Error In"=w119, "Alligator Queue Element 2"=w113, "Alligator Queue Element 1"=w120) -> ("Error Out"=w107:errorcluster, "Alligator Queue Element 1 (+ 2)"=w117:T2[])  [unwired: 6 in]
        n32 = Format Into String(format string="Calibrated Phasor Map Series Script (%d steps) started on %s at %s" ("initial string"), error in=w107, w109, w114, w115) -> (resulting string=w108:string, error out=w106:errorcluster)  [unwired: 1 in]
      }
    }
    n33 = Increment(x=w27) -> (x+1=w26:T5)
  }
  "Error Out" <- w6
  "Alligator Queue Elements out" <- w12
  "Series Length" <- w9
  "Message" <- w1
  n34 = call "Alligator Variables Storage.vi"("Get(F)/Set"=TRUE, "AlliGator Variable"=AlliGator_Variables_List."GUI:Script in progress" ("Alligator Variable"), "Error In"=w6, "Data in"=TRUE) -> ()  [unwired: 5 in, 3 out]
